vi "Compare_Costs_(11)_F()_Rearrange_Indices-1.vi"(5 "[IN] Cost functions":i8[](array[numeric]), 6 "[IN] # of Longest track\nInside the Tracks Group":i32, 7 "[IN] Subtracks":T1(array[cluster])) -> (2 "[OUT] Indicies of sub\ntracks for transforma\ntion (resolving)":i32[](array[numeric]))   [LabVIEW 2013]
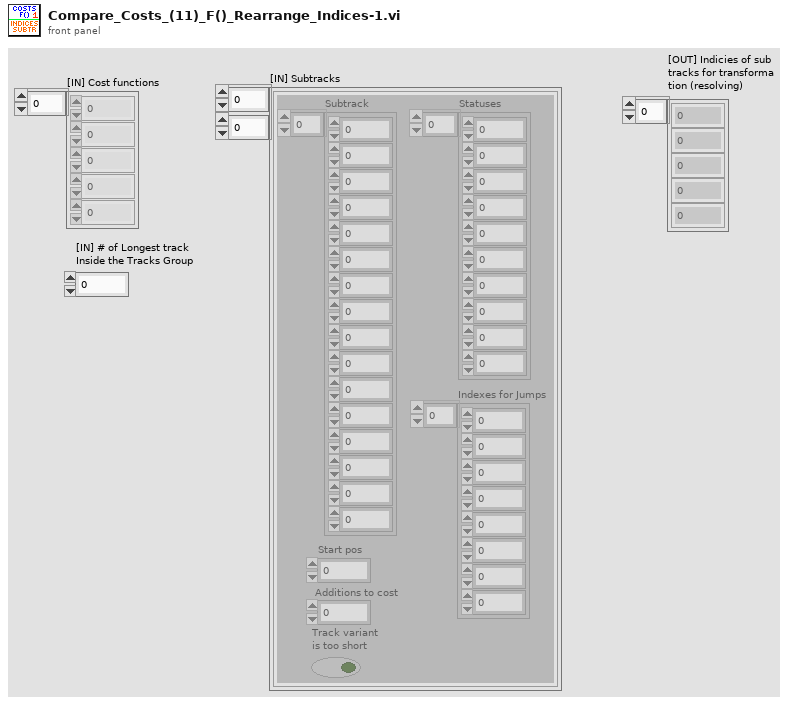
[diagram p1: front panel]
types:
  T1 = cluster{"Subtrack":dbl[], "Statuses":i16[], "Start pos":i32, "Additions to cost":i32, "Track variant \nis too short":bool, "Indexes for Jumps":i32[]}[][]
  T2 = cluster{"Subtrack":dbl[], "Statuses":i16[], "Start pos":i32, "Additions to cost":i32, "Track variant \nis too short":bool, "Indexes for Jumps":i32[]}
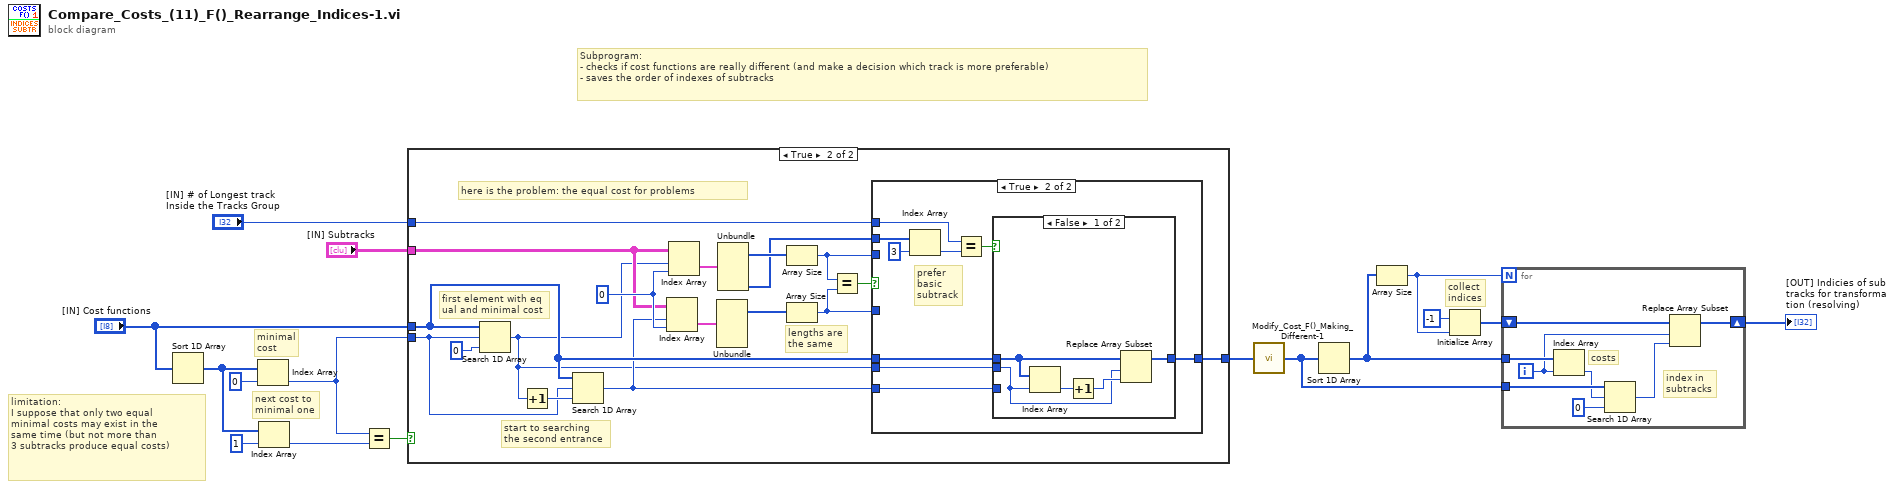
[diagram p0: block diagram]
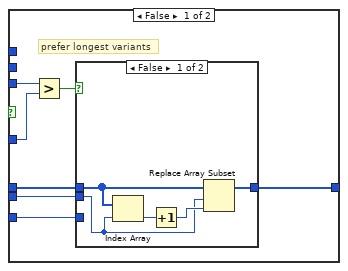
[diagram p3: hidden frame]
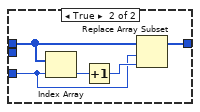
[diagram p4: hidden frame]
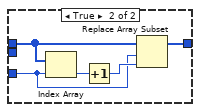
[diagram p5: hidden frame]
diagram:
  # "collect\nindices"
  # "limitation: \nI suppose that only two equal\nminimal costs may exist in the \nsame time (but not more than\n3 subtracks produce equal costs)"
  # "next cost to \nminimal one"
  # "minimal\ncost"
  # "Subprogram:\n- checks if cost functions are really different (and make a decision which track is more preferable)\n- saves the order of indexes of subtracks"
  n1 = Sort 1D Array(array="[IN] Cost functions") -> (sorted array=w11:i8[])
  n2 = Index Array(array=w11, index=0) -> (element=w10:i8)
  n3 = Index Array(array=w11, index=1) -> (element=w14:i8)
  n4 = Equal?(x=w10, y=w14) -> (x = y?=w13:bool)
  n5 = case shown="True" w13 {
    tunnel: "[IN] Subtracks" -> [_ w30]
    tunnel: "[IN] Cost functions" -> [w17 w23]
    tunnel: w10 -> [_ w33]
    tunnel: "[IN] # of Longest track\nInside the Tracks Group" -> [_ w25]
    tunnel: [w17 w18] -> w2
    frame False {
    }
    frame True {
      w31 = 0 ("disabled index (row)")
      # "lengths are\nthe same"
      # "start to searching\nthe second entrance"
      # "first element with eq\nual and minimal cost"
      # "here is the problem: the equal cost for problems"
      n6 = Search 1D Array(1D array=w23, element=w33, start index (0)=0) -> (index of element=w21:i32)
      n7 = Increment(x=w21) -> (x+1=w34:i32)
      n8 = Search 1D Array(1D array=w23, element=w33, start index (0)=w34) -> (index of element=w22:i32)
      n9 = Index Array(array=w30, index (row)=w22, index (col)=w31) -> (element=w29:T2)
      n10 = Index Array(array=w30, index (row)=w21, index (col)=w31) -> (element=w32:T2)
      n11 = Unbundle(w29) -> ("Statuses"=w27:i16[])  [unwired: 5 out]
      n12 = Unbundle(w32) -> ("Statuses"=w28:i16[], "Indexes for Jumps"=w24:i32[])  [unwired: 4 out]
      n13 = Array Size(array=w28) -> (size(s)=w20:i32)
      n14 = Array Size(array=w27) -> (size(s)=w19:i32)
      n15 = Equal?(x=w20, y=w19) -> (x = y?=w26:bool)
      n16 = case shown="True" w26 {
        tunnel: w25 -> [_ w59]
        tunnel: w24 -> [_ w61]
        tunnel: w23 -> [w39 w56]
        tunnel: [w36 w55] -> w18
        tunnel: w22 -> [w38 w54]
        tunnel: w21 -> [w37 w53]
        tunnel: w20 -> [w42 _]
        tunnel: w19 -> [w41 _]
        frame False {
          # "prefer longest variants"
          n17 = Greater?(x=w42, y=w41) -> (0:w40:bool)
          n18 = case shown="False" w40 {
            tunnel: w39 -> [w45 w51]
            tunnel: [w44 w49] -> w36
            tunnel: w38 -> [_ w48]
            tunnel: w37 -> [w43 _]
            frame False {
              n19 = Index Array(array=w45, index=w43) -> (element=w47:i8)
              n20 = Increment(x=w47) -> (x+1=w46:i8)
              n21 = Replace Array Subset(array=w45, new element=w46, index=w43) -> (w44:i8[])
            }
            frame True {
              n22 = Index Array(array=w51, index=w48) -> (element=w52:i8)
              n23 = Increment(x=w52) -> (x+1=w50:i8)
              n24 = Replace Array Subset(array=w51, new element=w50, index=w48) -> (w49:i8[])
            }
          }
        }
        frame True {
          # "prefer \nbasic \nsubtrack"
          n25 = Index Array(array=w61, index=3) -> (element=w58:i32)
          n26 = Equal?(x=w59, y=w58) -> (x = y?=w57:bool)
          n27 = case shown="False" w57 {
            tunnel: w56 -> [w64 w70]
            tunnel: [w63 w68] -> w55
            tunnel: w54 -> [_ w67]
            tunnel: w53 -> [w62 _]
            frame False {
              n28 = Index Array(array=w64, index=w62) -> (element=w66:i8)
              n29 = Increment(x=w66) -> (x+1=w65:i8)
              n30 = Replace Array Subset(array=w64, new element=w65, index=w62) -> (w63:i8[])
            }
            frame True {
              n31 = Index Array(array=w70, index=w67) -> (element=w71:i8)
              n32 = Increment(x=w71) -> (x+1=w69:i8)
              n33 = Replace Array Subset(array=w70, new element=w69, index=w67) -> (w68:i8[])
            }
          }
        }
      }
    }
  }
  n34 = call "Modify_Cost_F()_Making_Different-1.vi"("[IN] Cost functions"=w2) -> ("[OUT] Cost functions"=w1:i8[])
  n35 = Sort 1D Array(array=w1) -> (sorted array=w4:i8[])
  n36 = Array Size(array=w4) -> (size(s)=w6:i32)
  n37 = Initialize Array(-1 ("index"), w6) -> (w5:i32[])
  n38 = for {
    N: w6 -> [_]
    shift-right: [w73] -> w3
    shift-left: w5 -> [w75]
    tunnel: w4 -> [w79]
    tunnel: w1 -> [w78]
    i -> [w72]
    # "index in\nsubtracks"
    # "costs"
    n39 = Index Array(array=w79, index=w72) -> (element=w77:i8)
    n40 = Search 1D Array(1D array=w78, element=w77, start index (0)=0) -> (index of element=w74:i32)
    n41 = Replace Array Subset(array=w75, new element=w74, index=w72) -> (w73:i32[])
  }
  "[OUT] Indicies of sub\ntracks for transforma\ntion (resolving)" <- w3
